vi "Set Feeder.vi"(8 "error in (no error)":errorcluster, 9 "Component":enum16{"All", "Mixer", "Screw", "Solenoid"}(ring), 10 "State":bool, 11 "Feeder Actor.lvlib:Feeder.lvclass":refnum<class "Feeder.lvclass">) -> (0 "error out":errorcluster, 3 "Feeder Actor.lvlib:Feeder.lvclass 2":refnum<class "Feeder.lvclass">)   [LabVIEW 2018, in "Feeder Actor.lvlib" / "Feeder.lvclass"]
uses:
  Feeder.lvclass
  C:/Program Files/National Instruments/LabVIEW 2018/vi.lib/ActorFramework/Actor/Actor.lvclass
  <vilib>/ActorFramework/Actor/Actor.lvclass/Actor.ctl
  Feeder.lvclass/Feeder.ctl
  Solenoid Messages/Set Solonoid Msg/Set Solonoid Msg.lvclass/Set Solonoid Msg.ctl
  <vilib>/ActorFramework/Message Enqueuer/Message Enqueuer.lvclass/Message Enqueuer.ctl
  <vilib>/ActorFramework/Message Enqueuer/Enqueue.vi
  Solenoid Messages/Set Solonoid Msg/Set Solonoid Msg.lvclass
  C:/Program Files/National Instruments/LabVIEW 2018/vi.lib/ActorFramework/Message/Message.lvclass
  <vilib>/ActorFramework/Message Priority Queue/Priority Enqueue.vi
  Counter Messages/Print Msg/Print Msg.lvclass
  <vilib>/ActorFramework/Actor/Actor.lvclass
  ADM/Main Messages/Print Switch Finished Msg/Print Switch Finished Msg.lvclass
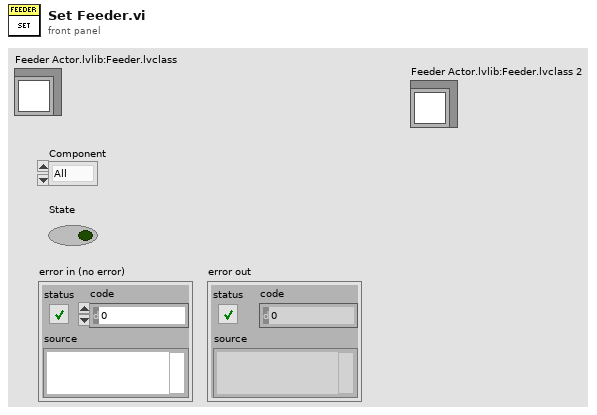
[diagram p1: front panel]
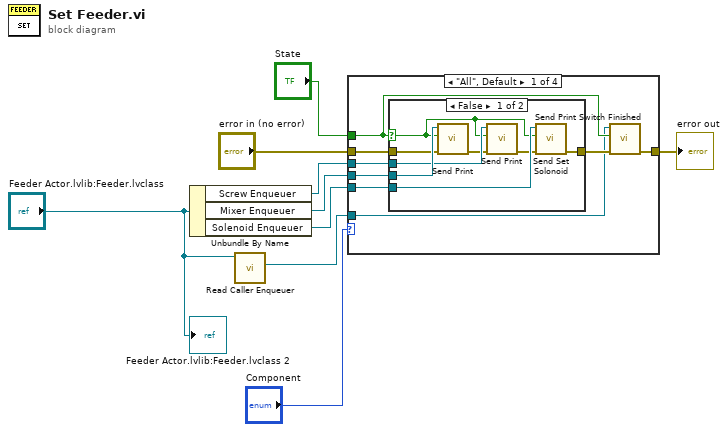
[diagram p0: block diagram]
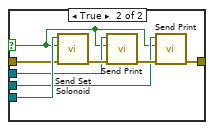
[diagram p2: hidden frame]
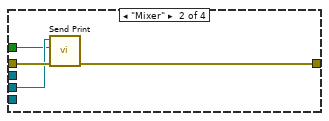
[diagram p3: hidden frame]
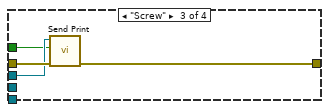
[diagram p4: hidden frame]
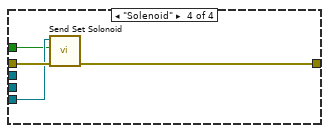
[diagram p5: hidden frame]
diagram:
  n1 = Unbundle By Name("Feeder Actor.lvlib:Feeder.lvclass") -> ("Screw Enqueuer"=w7:refnum<class "Message Enqueuer.lvclass">, "Mixer Enqueuer"=w8:refnum<class "Message Enqueuer.lvclass">, "Solenoid Enqueuer"=w9:refnum<class "Message Enqueuer.lvclass">)
  n2 = call <vilib>:"Read Caller Enqueuer.vi"("Actor"="Feeder Actor.lvlib:Feeder.lvclass") -> ("Caller Enqueuer"=w2:refnum<class "Message Enqueuer.lvclass">)  [unwired: 10 in]
  n3 = case shown="\"All\", Default" "Component" {
    tunnel: "State" -> [w12 w34 w38 w42]
    tunnel: w9 -> [w17 _ _ w43]
    tunnel: w8 -> [w16 w35 _ _]
    tunnel: w7 -> [w15 _ w39 _]
    tunnel: "error in (no error)" -> [w14 w36 w40 w45]
    tunnel: [w10 w37 w41 w44] -> w1
    tunnel: w2 -> [w11 _ _ _]
    frame "All", Default {
      n4 = case shown="False" w12 {
        selector: w12 -> [w18 w26]
        tunnel: w17 -> [w25 w33]
        tunnel: w16 -> [w23 w27]
        tunnel: w15 -> [w21 w30]
        tunnel: w14 -> [w22 w32]
        tunnel: [w24 w29] -> w13
        frame False {
          n5 = call "Send Print.vi"("error in (no error)"=w22, "On?"=w18, "Message Enqueuer in"=w23) -> ("error out"=w19:errorcluster)  [unwired: 7 in, 1 out]
          n6 = call "Send Print.vi"("error in (no error)"=w19, "On?"=w18, "Message Enqueuer in"=w21) -> ("error out"=w20:errorcluster)  [unwired: 7 in, 1 out]
          n7 = call "Send Set Solonoid.vi"("error in (no error)"=w20, "State"=w18, "Message Enqueuer in"=w25) -> ("error out"=w24:errorcluster)  [unwired: 7 in, 1 out]
        }
        frame True {
          n8 = call "Send Set Solonoid.vi"("error in (no error)"=w32, "State"=w26, "Message Enqueuer in"=w33) -> ("error out"=w31:errorcluster)  [unwired: 7 in, 1 out]
          n9 = call "Send Print.vi"("error in (no error)"=w31, "On?"=w26, "Message Enqueuer in"=w30) -> ("error out"=w28:errorcluster)  [unwired: 7 in, 1 out]
          n10 = call "Send Print.vi"("error in (no error)"=w28, "On?"=w26, "Message Enqueuer in"=w27) -> ("error out"=w29:errorcluster)  [unwired: 7 in, 1 out]
        }
      }
      n11 = call "Send Print Switch Finished.vi"("error in (no error)"=w13, "State"=w12, "Message Enqueuer in"=w11) -> ("error out"=w10:errorcluster)  [unwired: 7 in, 1 out]
    }
    frame "Mixer" {
      n12 = call "Send Print.vi"("error in (no error)"=w36, "On?"=w34, "Message Enqueuer in"=w35) -> ("error out"=w37:errorcluster)  [unwired: 7 in, 1 out]
    }
    frame "Screw" {
      n13 = call "Send Print.vi"("error in (no error)"=w40, "On?"=w38, "Message Enqueuer in"=w39) -> ("error out"=w41:errorcluster)  [unwired: 7 in, 1 out]
    }
    frame "Solenoid" {
      n14 = call "Send Set Solonoid.vi"("error in (no error)"=w45, "State"=w42, "Message Enqueuer in"=w43) -> ("error out"=w44:errorcluster)  [unwired: 7 in, 1 out]
    }
  }
  "error out" <- w1
  "Feeder Actor.lvlib:Feeder.lvclass 2" <- "Feeder Actor.lvlib:Feeder.lvclass"
